vi "Arm Acceleration Limitation.vi"(8 "Max Change":dbl, 11 "Input":dbl) -> (3 "New Speed":dbl)   [LabVIEW 2014]
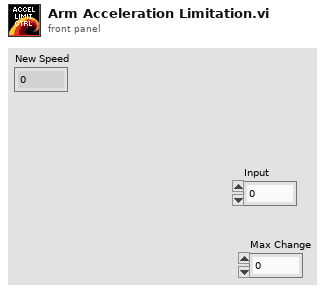
[diagram p1: front panel]
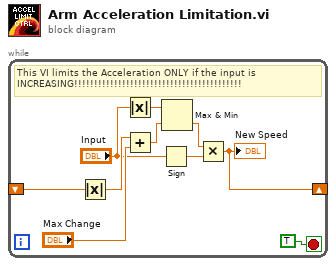
[diagram p0: block diagram]
diagram:
  n1 = while {
    shift-right: [w2] -> _
    shift-left: _ -> [w4]
    stop <- TRUE stop-if-true
    # "This VI limits the Acceleration ONLY if the input is\nINCREASING!!!!!!!!!!!!!!!!!!!!!!!!!!!!!!!!!!!!!!!!!!"
    n2 = Absolute Value(x=w4) -> (abs(x)=w5:dbl)
    n3 = Absolute Value(x="Input") -> (abs(x)=w8:dbl)
    n4 = Add(x=w5, y="Max Change") -> (x+y=w7:dbl)
    n5 = Sign(1:"Input") -> (0:w10:dbl)
    n6 = Max & Min(x=w8, y=w7) -> (min(x,y)=w9:dbl)  [unwired: 1 out]
    n7 = Multiply(x=w9, y=w10) -> (x*y=w2:dbl)
    "New Speed" <- w2
  }
